vi "RT Globals RD v1.0.vi"() -> ()   [LabVIEW 2019]
panel:
  out "Xsens INS Data Out":string[][](array[string])
  in  "Kill System Messenger":bool
  out "Xsens GNSS Data Out":string[][](array[string])
  in  "Packet 20 Decoded Data Cluster 2":T1
  out "Uptime":string
  out "Heading":string
  out "Offset Distance":string
  out "Current Position":string
  out "PTP TimeKeeper Detected":bool
  out "SD System Status":bool[](array[boolean])
  out "SD Filter Status":bool[](array[boolean])
  out "Spatial Dual Timestamp (External)":u64
  out "Enable Sys Clock Update":bool
  out "satellites available":u8
  out "GNSS Fix Status":u32
  out "1 Hz INS Out":dbl[](array[numeric])
  in  "Global Stop":bool
  out "Separation Distance":dbl
  out "Current Longitude":dbl
  out "Current Latitude":dbl
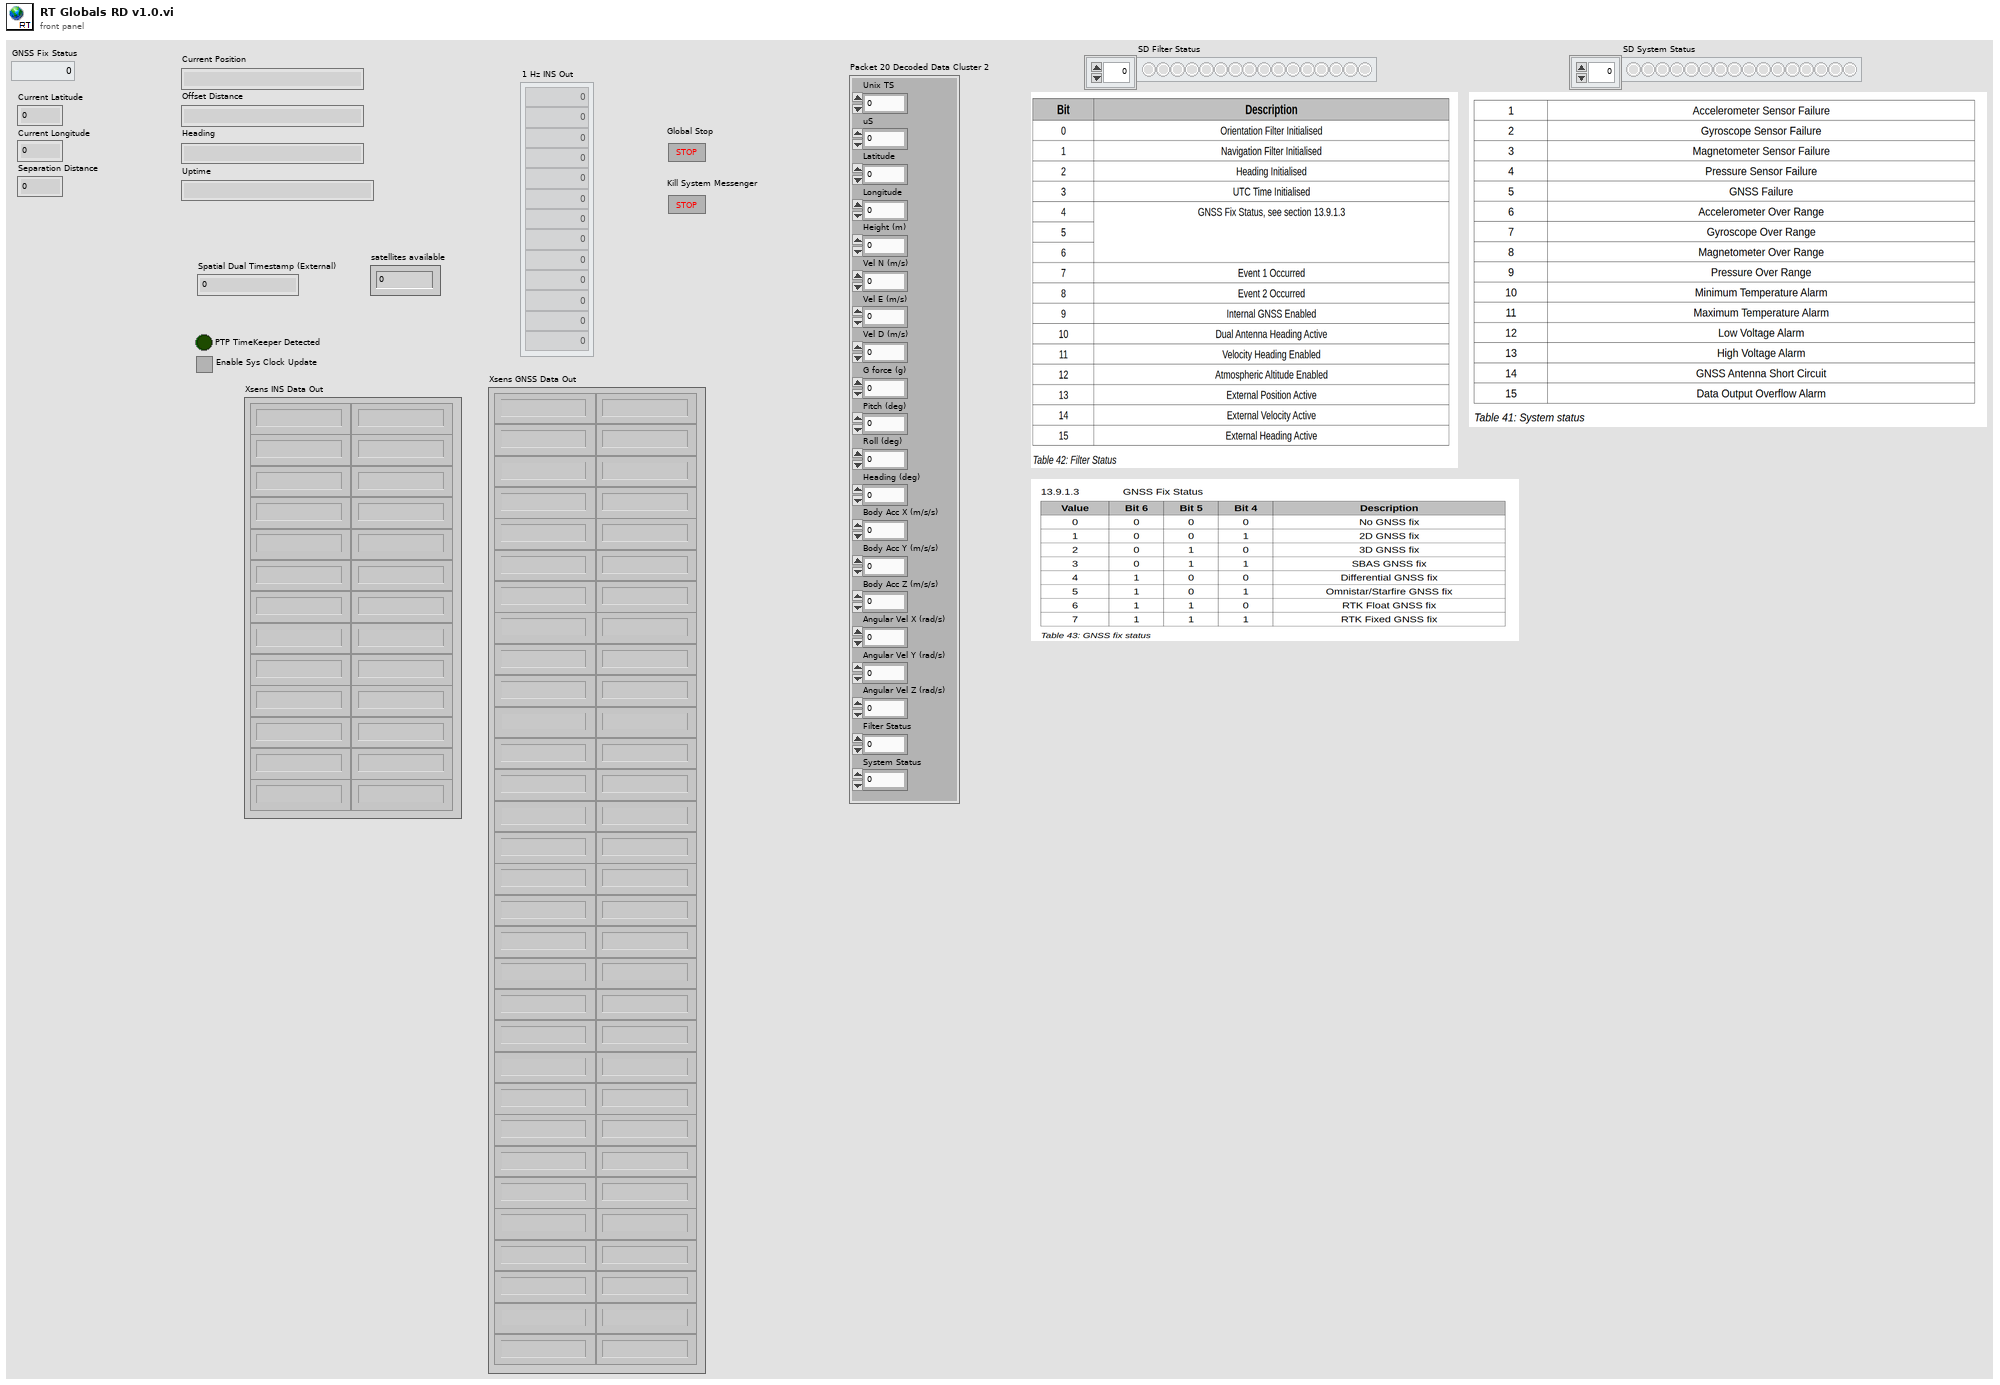
[diagram p1: front panel]
types:
  T1 = cluster{"Unix TS":u32, "uS":u32, "Latitude":dbl, "Longitude":dbl, "Height (m)":dbl, "Vel N (m/s)":sgl, "Vel E (m/s)":sgl, "Vel D (m/s)":sgl, "G force (g)":sgl, "Pitch (deg)":sgl, "Roll (deg)":sgl, "Heading (deg)":sgl, "Body Acc X (m/s/s)":sgl, "Body Acc Y (m/s/s)":sgl, "Body Acc Z (m/s/s)":sgl, "Angular Vel X (rad/s)":sgl, "Angular Vel Y (rad/s)":sgl, "Angular Vel Z (rad/s)":sgl, "Filter Status":u16, "System Status":u16}
diagram:
